vi "Process File.vi"(8 "error in (no error)":errorcluster, 10 "File":path, 11 "Integrate in":refnum<class "Integrate.lvclass">) -> (0 "error out":errorcluster, 2 "File out":path, 3 "Integrate out":refnum<class "Integrate.lvclass">)   [LabVIEW 2016, in "Integrate.lvclass"]
uses:
  Integrate.lvclass
  C:/Program Files/National Instruments/LabVIEW 2016/vi.lib/ActorFramework/Actor/Actor.lvclass
  <vilib>/ActorFramework/Actor/Actor.lvclass/Actor.ctl
  Channel peak.ctl
  Monitor-Pulse Messages/Write Peak Field Msg/Write Peak Field Msg.lvclass/Write Peak Field Msg.ctl
  <vilib>/ActorFramework/Message Enqueuer/Message Enqueuer.lvclass/Message Enqueuer.ctl
  <vilib>/ActorFramework/Message Enqueuer/Enqueue.vi
  Monitor-Pulse Messages/Write Peak Field Msg/Write Peak Field Msg.lvclass
  C:/Program Files/National Instruments/LabVIEW 2016/vi.lib/ActorFramework/Message/Message.lvclass
  Read Integrate Configuration.vi
  <vilib>/ActorFramework/Message Priority Queue/Priority Enqueue.vi
  <vilib>/ActorFramework/Actor/Actor.lvclass
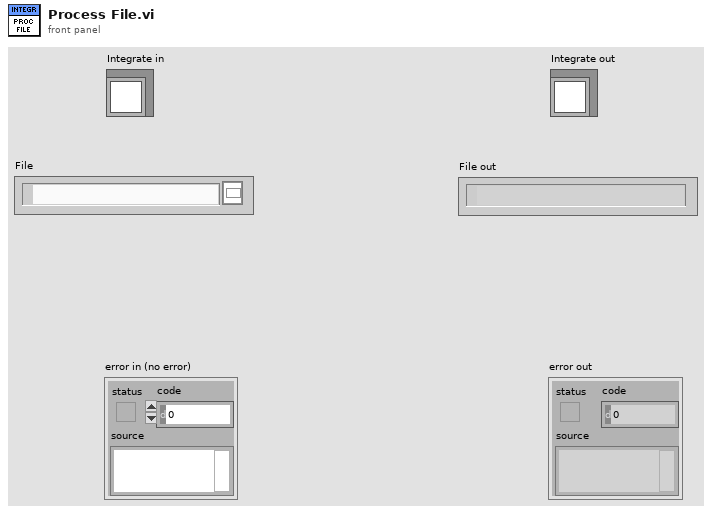
[diagram p1: front panel]
types:
  T1 = typedef "Integrator Configoration.ctl" = cluster{"Integrate":T2[], "Offset duration ":dbl, "TDMS group name":string}
  T2 = typedef "Integrate channel.ctl" = cluster{"Channel":string, "Output name":string, "Factor":dbl, "Start time":dbl, "Duration":dbl}
  T3 = typedef "Channel peak.ctl" = cluster{"Peak":dbl, "Name":string}
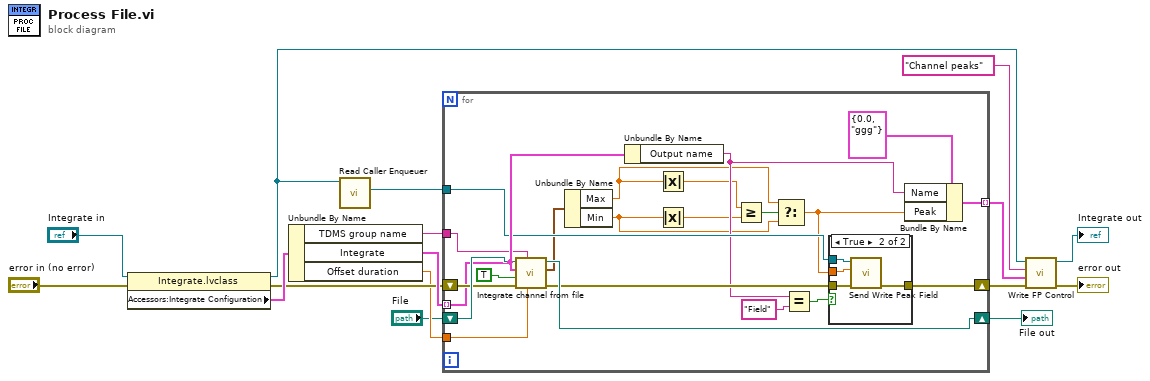
[diagram p0: block diagram]
diagram:
  n1 = property class="Integrate.lvclass"(reference="Integrate in", error in="error in (no error)") -> (reference out=w6:refnum<class "Integrate.lvclass">, error out=w13:errorcluster, "Accessors:Integrate Configuration"=w15:T1)
  n2 = Unbundle By Name(w15) -> ("TDMS group name"=w10:string, "Integrate"=w14:T2[], "Offset duration"=w12:dbl)
  n3 = call <vilib>:"Read Caller Enqueuer.vi"("Actor"=w6) -> ("Caller Enqueuer"=w11:refnum<class "Message Enqueuer.lvclass">)  [unwired: 10 in]
  n4 = for {
    tunnel: w14 -> [w33] mode=indexing
    shift-right: [w37] -> w7
    shift-left: "File" -> [w38]
    tunnel: w12 -> [w34]
    shift-right: [w29] -> w4
    shift-left: w13 -> [w35]
    tunnel: w11 -> [w28]
    tunnel: w10 -> [w27]
    tunnel: [w17] -> w2 mode=indexing
    n5 = call "Integrate channel from file.vi"("Offset duration"=w34, "group name in"=w27, "Error In"=w35, "Save data"=TRUE, "Integration settings"=w33, "File Path Control"=w38) -> ("Error Out"=w30:errorcluster, "Min max"=w19:cluster{"Max":dbl, "Min":dbl}, "File Path out"=w37:path)  [unwired: 2 in, 1 out]
    n6 = Unbundle By Name(w19) -> ("Max"=w21:dbl, "Min"=w24:dbl)
    n7 = Unbundle By Name(w33) -> ("Output name"=w25:string)
    n8 = Absolute Value(x=w21) -> (abs(x)=w22:dbl)
    n9 = Absolute Value(x=w24) -> (abs(x)=w23:dbl)
    n10 = Greater Or Equal?(x=w22, y=w23) -> (x >= y?=w20:bool)
    n11 = Select(t=w21, s=w20, f=w24) -> (s? t:f=w18:dbl)
    n12 = Equal?(x=w25, y="Field") -> (x = y?=w31:bool)
    n13 = case shown="True" w31 {
      tunnel: w30 -> [w39 w43]
      tunnel: [w39 w42] -> w29
      tunnel: w28 -> [_ w41]
      tunnel: w18 -> [_ w40]
      frame False {
      }
      frame True {
        n14 = call "Send Write Peak Field.vi"("error in (no error)"=w43, "Peak Field"=w40, "Message Enqueuer"=w41) -> ("error out"=w42:errorcluster)  [unwired: 7 in, 1 out]
      }
    }
    n15 = Bundle By Name(cluster=T3 {"Peak"=0.0, "Name"="ggg"} ("Channel peak"), "Name"=w25, "Peak"=w18) -> (w17:T3)
  }
  "File out" <- w7
  n16 = call-dynamic "Write FP Control.vi"("error in (no error)"=w4, "Control Value"=w2, "Control Name"="Channel peaks", "Measure Object in"=w6) -> ("error out"=→"error out":errorcluster, "Measure Object out"=→"Integrate out":refnum<class "Integrate.lvclass">)  [unwired: 6 in]
